vi "ControladorPIDparaSEIG.vi"() -> ()   [LabVIEW 2019]
uses:
  <resource>/objmgr/daqmx.rc
  <vilib>/addons/control/pid/NI_PID_pid.lvlib
  <vilib>/NI/Modbus Library/API/Wrapper/API Main.lvlib
  <vilib>/NI/Modbus Library/API/Master/Modbus Master.lvclass
  <vilib>/NI/Modbus Library/API/Wrapper/Create Serial Master.vi
  <vilib>/DAQmx/configure/timing.llb/DAQmx Timing (Sample Clock).vi
  <vilib>/DAQmx/create/channels.llb/DAQmx Create Channel (AI-Voltage-Basic).vi
  <vilib>/DAQmx/read.llb/DAQmx Read (Analog 2D DBL NChan NSamp).vi
  <vilib>/addons/control/pid/pid.llb/PID (DBL).vi
panel:
  in  "Tab Control":enum32{"Configuracion", "Datos"}(tab)=enum."Datos"
  in  "Valor máximo en la entrada":dbl=5.0 format="%0.2f"
  in  "Valor mínimo en la entrada":dbl=-5.0 format="%0.2f"
  in  "Modo de muestreo":i32(ring)=10123 items=["Finite Samples"=10178, "Continuous Samples"=10123, "Hardware Timed Single Point"=12522]
  in  "Muestras por canal":i32=500
  in  "Frecuencia de muetreo":dbl=2000.0 format="%0.2f"
  in  "VISA resource name":refnum<visa-resource-name>="COM3"
  in  "baud rate":u32=9600
  in  "unit ID":u8=17
  in  "physical channels":tag="myDAQ2/ai1, myDAQ2/ai0 "
  in  "number of samples per channel":i32=500
  out "dt out (s)":dbl=1e-05 format="%.3f"
  out "# pending remove":i32
  out "Ajuste VFD\n(Hz)":dbl=40.0 format="%#_4f"
  out "Voltage medido \n(Vrms)":dbl=0.3833916457369924 format="%#_4f"
  out "Actual Sample Rate":dbl=2000.0
  in  "Voltaje deseado\n(Vrms)":dbl=145.0 step=10.0
  in  "PID constantes":T1={"proportional gain (Kc)"=0.08, "integral time (Ti, min)"=0.0, "derivative time (Td, min)"=0.0} {"derivative time (Td, min)" format="%.3f"; "integral time (Ti, min)" format="%.3f"; "proportional gain (Kc)" format="%.3f"}
  out "Salida PID":dbl=5.0 format="%.2f"
  in  "Stop":bool
  out "Corriente Medida\n(Irms)":dbl=0.3833916457369924 format="%#_4f"
  out "Velocidad\nmedida (rpm)":i32
  out "Tension":cluster{"Vd":dbl, dbl}(graph) caption="Waveform Chart"
  out "Corriente":dbl(graph) caption="Waveform Chart"
  out "Velocidad":dbl(graph) caption="Waveform Chart"
  # "Modbus"
  # "Generador"
  # "Counter"
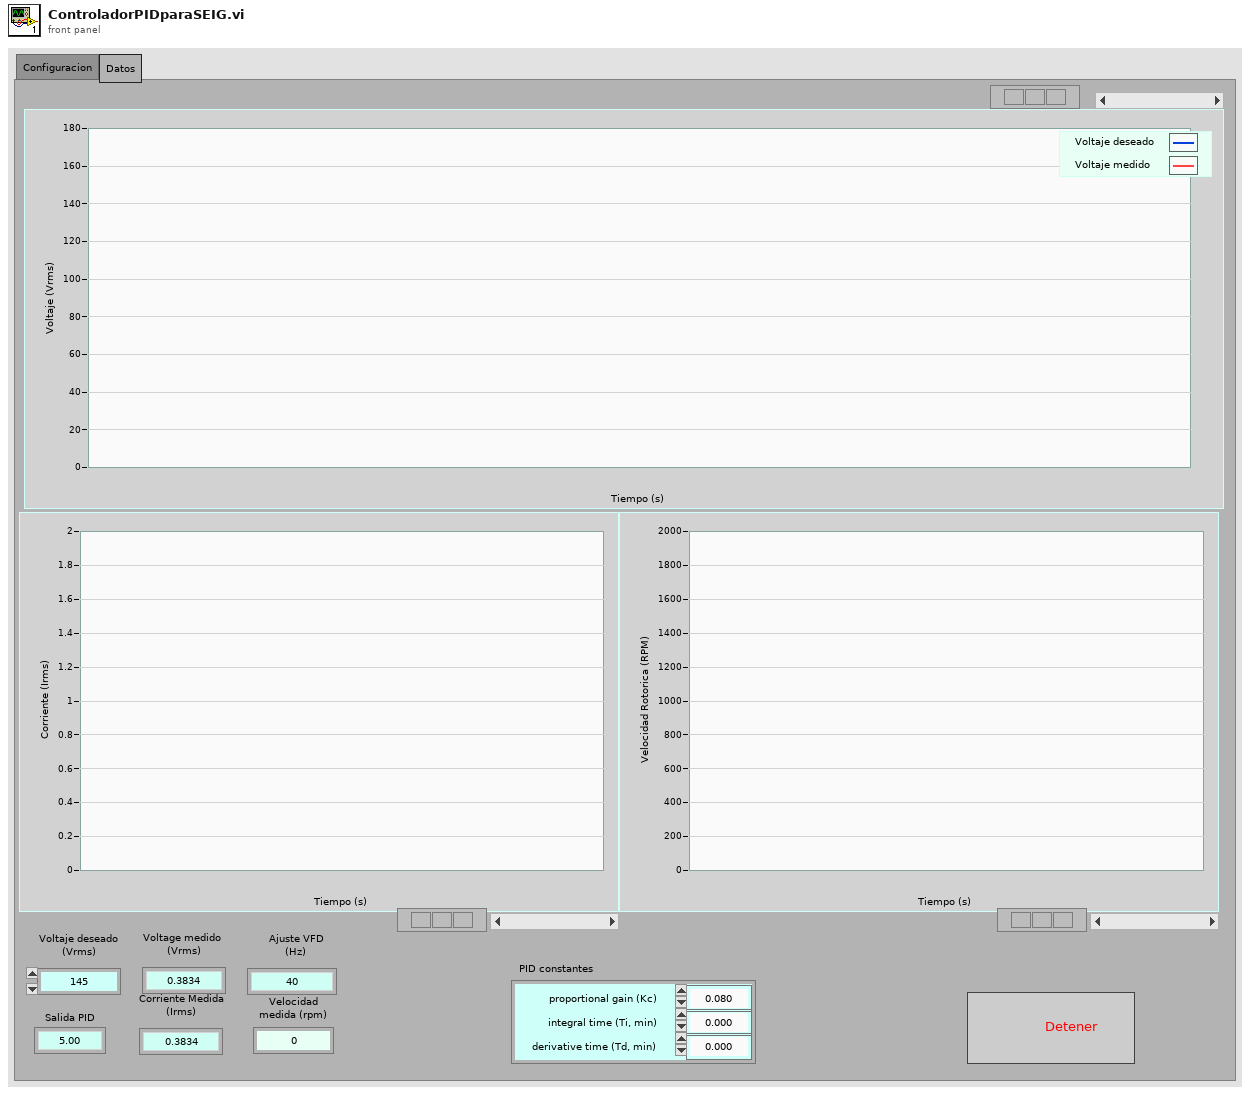
[diagram p1: front panel]
types:
  T1 = cluster{"proportional gain (Kc)":dbl, "integral time (Ti, min)":dbl, "derivative time (Td, min)":dbl}
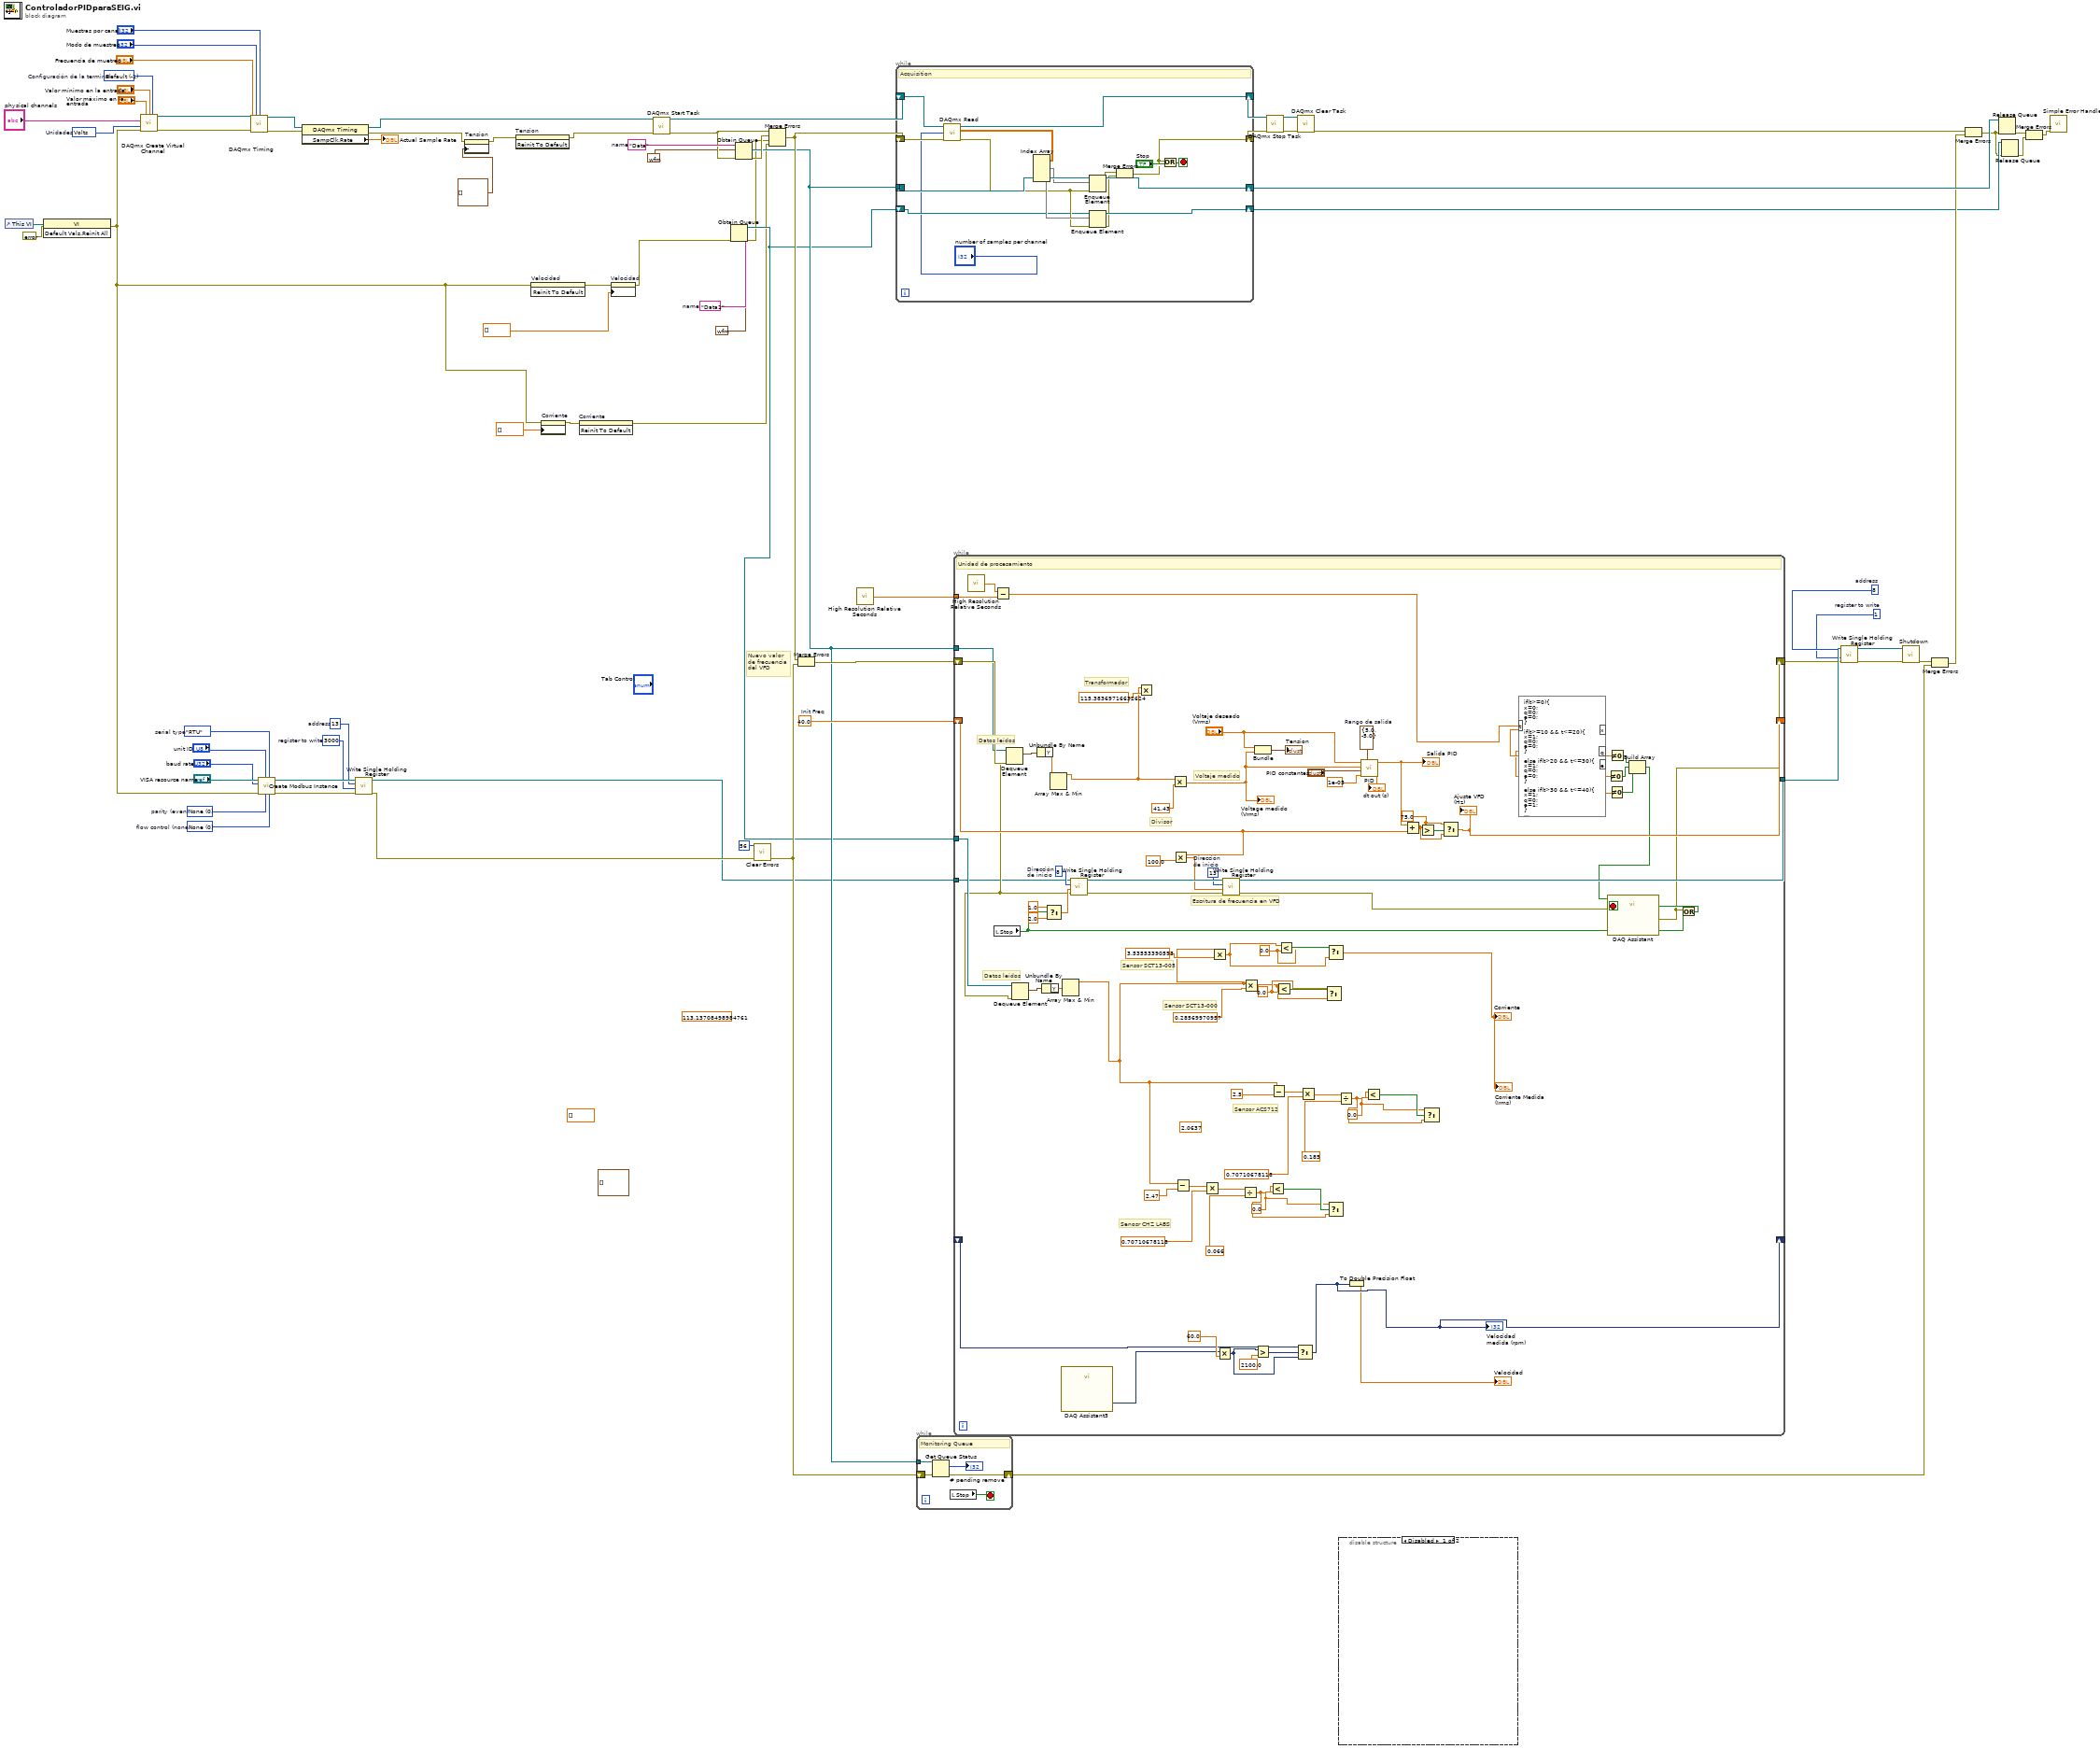
[diagram p0: block diagram]
diagram:
  (unwired) 113.13708498984761 ("y")
  (unwired) cluster{"Voltaje\ndeseado (Vrms)":dbl, dbl}[] [] ("History Data")
  (unwired) dbl[] [] ("History Data")
  w21 = "Data1"  # name
  w24 = u16 1  # register to write
  w25 = u16 8  # address
  w41 = u16 3000  # register to write
  w42 = u16 13  # address
  w47 = u16 0 items=["None", "XON/XOFF", "RTS/CTS", "XON/XOFF & RTS/CTS", "DTR/DSR", "XON/XOFF & DTR/DSR"]  # flow control (none)
  w48 = u16 0 items=["None", "Odd", "Even", "Mark", "Space"]  # parity (even)
  w49 = enum16{"RTU", "ASCII"}."RTU"  # serial type
  w52 = 40.0  # Init Freq
  w59 = "Data"  # name
  w72 = -1 items=["Default"=-1, "RSE"=10083, "NRSE"=10078, "Differential"=10106, "Pseudodifferential"=12529]  # Configuración de la terminal
  w75 = 10348 items=["Volts"=10348, "From Custom Scale"=10065]  # Unidades
  # "Nuevo valor\nde frecuencia\ndel VFD"
  n1 = control-ref of="This VI"() -> (w32:refnum<vi>)
  n2 = invoke class="VI" method="Default Vals.Reinit All"(reference=w32, error in=errorcluster {"status"=FALSE, "code"=0, "source"=""} ("error constant")) -> (error out=w7:errorcluster)  [unwired: 1 in, 2 out]
  n3 = call-poly <vilib>:"DAQmx Create Virtual Channel.vi"("maximum value"="Valor máximo en la entrada", "minimum value"="Valor mínimo en la entrada", "input terminal configuration"=w72, "physical channels"="physical channels", "units"=w75, "error in"=w7) -> ("task out"=w70:refnum<k21>, "error out"=w71:errorcluster)  [unwired: 8 in]
  n4 = call-poly <vilib>:"DAQmx Timing.vi"("task/channels in"=w70, "sample mode"="Modo de muestreo", "samples per channel"="Muestras por canal", "rate"="Frecuencia de muetreo", "error in"=w71) -> ("task out"=w61:refnum<k21>, "error out"=w60:errorcluster)  [unwired: 9 in]
  n5 = call-poly <vilib>:"Create Modbus Instance.vi"("flow control (none)"=w47, "serial type"=w49, "parity (even)"=w48, "unit ID"="unit ID", "error in"=w7, "baud rate"="baud rate", "VISA resource name"="VISA resource name") -> ("error out"=w44:errorcluster, "serial master instance"=w43:refnum<class "Modbus Master.lvclass">)  [unwired: 3 in]
  n6 = property class="DAQmx Timing"(reference=w61, error in=w60) -> (reference out=w23:refnum<k21>, error out=w3:errorcluster, "SampClk.Rate"=→"Actual Sample Rate":dbl)
  n7 = call-dynamic "Write Single Holding Register.vi"("error in"=w44, "register to write"=w41, "address"=w42, "Modbus master in"=w43) -> ("error out"=w2:errorcluster, "Modbus master out"=w1:refnum<class "Modbus Master.lvclass">)  [unwired: 6 in]
  n8 = property on="Tension" class="WFChart (strict)"(error in=w3, "History Data"=cluster{"Voltaje\ndeseado (Vrms)":dbl, dbl}[] []) -> (error out=w5:errorcluster)  [unwired: 1 in, 1 out]
  n9 = invoke on="Tension" class="WFChart (strict)" method="Reinit To Default"(error in=w5) -> (error out=w4:errorcluster)  [unwired: 2 in, 2 out]
  n10 = invoke on="Velocidad" class="WFChart (strict)" method="Reinit To Default"(error in=w7) -> (error out=w14:errorcluster)  [unwired: 2 in, 2 out]
  n11 = property on="Corriente" class="WFChart (strict)"(error in=w7, "History Data"=dbl[] []) -> (error out=w10:errorcluster)  [unwired: 1 in, 1 out]
  n12 = invoke on="Corriente" class="WFChart (strict)" method="Reinit To Default"(error in=w10) -> (error out=w9:errorcluster)  [unwired: 2 in, 2 out]
  n13 = property on="Velocidad" class="WFChart (strict)"(error in=w14, "History Data"=dbl[] []) -> (error out=w12:errorcluster)  [unwired: 1 in, 1 out]
  n14 = call <vilib>:"DAQmx Start Task.vi"("task/channels in"=w23, "error in"=w4) -> ("task out"=w67:refnum<k21>, "error out"=w58:errorcluster)  [unwired: 12 in]
  n15 = Obtain Queue(name (unnamed)=w21, element data type=waveform(dbl) {"t0"=timestamp(0 s since 1904-01-01), "dt"=0.0, "Y"=[]} ("data"), error in (no error)=w12) -> (queue out=w18:refnum<queue>, error out=w8:errorcluster)  [unwired: 2 in, 1 out]
  n16 = Obtain Queue(name (unnamed)=w59, element data type=waveform(dbl) {"t0"=timestamp(0 s since 1904-01-01), "dt"=0.0, "Y"=[]} ("data"), error in (no error)=w58) -> (queue out=w37:refnum<queue>, error out=w57:errorcluster)  [unwired: 2 in, 1 out]
  n17 = call <vilib>:"Clear Errors.vi"("error in (no error)"=w2, "specific error code to clear (0: all)"=56) -> ("error out"=w34:errorcluster)  [unwired: 4 in, 1 out]
  n18 = Merge Errors(w58, w57, w8, w9) -> (w56:errorcluster)
  n19 = Merge Errors(w56, w34) -> (w45:errorcluster)
  n20 = call <vilib>:"High Resolution Relative Seconds.vi"() -> ("relative seconds"=w22:dbl)
  n21 = while {
    shift-right: [w77] -> w64
    shift-left: w56 -> [w91]
    shift-right: [w89] -> w63
    shift-left: w67 -> [w90]
    tunnel: w37 -> [w88]
    shift-right: [w87] -> w38
    shift-left: _ -> [_]
    shift-right: [w80] -> w16
    shift-left: w18 -> [w81]
    stop <- w92 stop-if-true
    # "Acquisition"
    n22 = call-poly <vilib>:"DAQmx Read.vi"("task/channels in"=w90, "number of samples per channel"="number of samples per channel", "error in"=w91) -> ("task out"=w89:refnum<k21>, "data"=w85:dbl[][], "error out"=w82:errorcluster)  [unwired: 10 in]
    n23 = Index Array(array=w85) -> (element #1=w84:dbl[], element #2=w83:dbl[])  [unwired: 4 in]
    n24 = Enqueue Element(queue=w88, element=w84, error in (no error)=w82) -> (queue out=w87:refnum<queue>, error out=w79:errorcluster)  [unwired: 1 in, 1 out]
    n25 = Enqueue Element(queue=w81, element=w83, error in (no error)=w82) -> (queue out=w80:refnum<queue>, error out=w78:errorcluster)  [unwired: 1 in, 1 out]
    n26 = Merge Errors(w79, w78) -> (w77:errorcluster)
    n27 = Or(x=w77, y="Stop") -> (x .or. y?=w92:bool)
  }
  n28 = while {
    tunnel: w37 -> [w96]
    shift-right: [w94] -> w35
    shift-left: w34 -> [w97]
    stop <- w93 stop-if-true
    # "Monitoring Queue"
    n29 = Get Queue Status(queue=w96, error in (no error)=w97) -> (# pending remove=→"# pending remove":i32, error out=w94:errorcluster)  [unwired: 1 in, 6 out]
    n30 = local read "Stop"() -> (w93:bool)
  }
  n31 = while {
    tunnel: w37 -> [w179]
    shift-right: [w153] -> w28
    shift-left: w45 -> [w180]
    shift-right: [w157] -> _
    shift-left: w52 -> [w144]
    tunnel: [w164] -> w29
    tunnel: w22 -> [w146]
    tunnel: w18 -> [w141]
    shift-right: [w134] -> _
    shift-left: _ -> [w133]
    tunnel: w1 -> [w102]
    stop <- w172 stop-if-true
    w114 = 0.0 ("y")
    w123 = 0.0 ("y")
    w127 = 0.0 ("y")
    (unwired) 2.0637 ("y")
    w107 = 0.0 ("y")
    w156 = 75.0 ("y")
    w166 = u16 13  # Dirección de inicio
    w169 = u16 8  # Dirección de inicio
    w177 = cluster{"output high":dbl, "output low":dbl} {"output high"=5.0, "output low"=-5.0}  # Rango de salida
    # "Divisor"
    # "Transformador"
    # "Sensor ACS712"
    # "Senosr CHZ LABS"
    # "Sensor SCT13-005"
    # "Sensor SCT13-000"
    # "Datos leídos"
    # "Escritura de frecuencia en VFD"
    # "Voltaje medido"
    # "Datos leídos"
    # "Unidad de procesamiento"
    n32 = call <vilib>:"High Resolution Relative Seconds.vi"() -> ("relative seconds"=w147:dbl)
    n33 = local read "Stop"() -> (w171:bool)
    n34 = Subtract(x=w147, y=w146) -> (x-y=w145:dbl)
    n35 = Dequeue Element(queue=w179, error in (no error)=w180) -> (element=w163:waveform(dbl), error out=w140:errorcluster)  [unwired: 1 in, 2 out]
    n36 = Dequeue Element(queue=w141, error in (no error)=w140) -> (element=w142:waveform(dbl))  [unwired: 1 in, 3 out]
    n37 = Unbundle By Name(w163) -> ("Y"=w176:dbl[])
    n38 = Unbundle By Name(w142) -> ("Y"=w143:dbl[])
    n39 = Select(t=1.0, s=w171, f=2.0 ("t")) -> (s? t:f=w170:dbl)
    n40 = Array Max & Min(array=w176) -> (max value=w98:dbl)  [unwired: 3 out]
    n41 = call "DAQ Assistant3"() -> ("data"=w135:dynamicdata)  [unwired: 17 in, 2 out]
    n42 = Array Max & Min(array=w143) -> (max value=w101:dbl)  [unwired: 3 out]
    n43 = call-dynamic "Write Single Holding Register.vi"("error in"=w140, "register to write"=w170, "address"=w169, "Modbus master in"=w102) -> ("error out"=w167:errorcluster, "Modbus master out"=w168:refnum<class "Modbus Master.lvclass">)  [unwired: 6 in]
    n44 = Multiply(x=w98, y=115.38369716632624) -> ()  [unwired: 1 out]
    n45 = Multiply(x=w98, y=41.43) -> (x*y=w175:dbl)
    "Voltage medido \n(Vrms)" <- w175
    n46 = Multiply(x=w144, y=100.0) -> (x*y=w165:dbl)
    n47 = Subtract(x=w101, y=2.47) -> (x-y=w111:dbl)
    n48 = Multiply(x=w111, y=0.70710678118) -> (x*y=w110:dbl)
    n49 = Multiply(x=w101, y=3.53553390593) -> (x*y=w106:dbl)
    n50 = Multiply(x=w135, y=60.0) -> (x*y=w136:dynamicdata)
    n51 = call-dynamic "Write Single Holding Register.vi"("error in"=w167, "register to write"=w165, "address"=w166, "Modbus master in"=w168) -> ("error out"=w154:errorcluster, "Modbus master out"=w164:refnum<class "Modbus Master.lvclass">)  [unwired: 6 in]
    n52 = Divide(x=w110, y=0.066) -> (x/y=w108:dbl)
    n53 = Multiply(x=w101, y=0.28569970957) -> (x*y=w125:dbl)
    n54 = Bundle("Voltaje deseado\n(Vrms)"="Voltaje deseado\n(Vrms)", w175) -> (→"Tension":cluster{"Voltaje deseado\n(Vrms)":dbl, dbl})  [unwired: 1 in]
    n55 = Greater?(x=w136, y=2100.0) -> (0:w132:dynamicdata)
    n56 = Less?(x=w108, y=w114) -> (x < y?=w115:bool)
    n57 = Subtract(x=w101, y=2.5) -> (x-y=w120:dbl)
    n58 = Less?(x=w125, y=w127) -> (x < y?=w128:bool)
    n59 = Less?(x=w106, y=w107) -> (x < y?=w131:bool)
    n60 = Select(t=w133, s=w132, f=w136) -> (s? t:f=w134:dynamicdata)
    "Velocidad\nmedida (rpm)" <- w134
    n61 = Multiply(x=w120, y=0.70710678118) -> (x*y=w119:dbl)
    n62 = Select(t=w127, s=w128, f=w125) -> ()  [unwired: 1 out]
    n63 = Select(t=w107, s=w131, f=w106) -> (s? t:f=→"Corriente Medida\n(Irms)" →"Corriente":dbl)
    n64 = Select(t=w114, s=w115, f=w108) -> ()  [unwired: 1 out]
    n65 = Divide(x=w119, y=0.185) -> (x/y=w117:dbl)
    n66 = To Double Precision Float(number=w134) -> (double precision float=→"Velocidad":dbl)
    n67 = call-poly <vilib>:"PID.vi"("output range"=w177, "dt (s)"=1e-05, "PID gains"="PID constantes", "process variable"=w175, "setpoint"="Voltaje deseado\n(Vrms)") -> ("dt out (s)"=→"dt out (s)":dbl, "output"=w178:dbl)  [unwired: 5 in]
    "Salida PID" <- w178
    n68 = Less?(x=w117, y=w123) -> (x < y?=w124:bool)
    n69 = Add(x=w178, y=w144) -> (x+y=w155:dbl)
    n70 = Greater?(x=w155, y=w156) -> (0:w158:bool)
    n71 = Select(t=w123, s=w124, f=w117) -> ()  [unwired: 1 out]
    n72 = Select(t=w156, s=w158, f=w155) -> (s? t:f=w157:dbl)
    "Ajuste VFD\n(Hz)" <- w157
    n73 = formula code="if(t>=0){\nx=0;\nq=0;\ne=0;\n}\n\nif(t>=10 && t<=20){\nx=1;\nq=0;\ne=0;\n}\n\nelse if(t>20 && t<=30){\nx=1;\nq=0;\ne=0;\n}\n\nelse if(t>30 && t<=40){\nx=1;\nq=0;\ne=1;\n}\n\nelse if(t>40 && t<=50){\nx=0;\nq=0;\ne=1;\n}\n\nelse{\nx=0;\nq=0;\ne=1;\n}"("t"=w145) -> ("x"=w152:dbl, "q"=w151:dbl, "e"=w103:dbl)
    n74 = Not Equal To 0?(x=w151) -> (x != 0?=w149:bool)
    n75 = Not Equal To 0?(x=w103) -> (x != 0?=w104:bool)
    n76 = Not Equal To 0?(x=w152) -> (x != 0?=w150:bool)
    n77 = Build Array(w150, w149, w104) -> (w148:bool[])
    n78 = call "DAQ Assistant"("data"=w148, "error in"=w154) -> ("error out"=w153:errorcluster)  [unwired: 16 in, 1 out]
    n79 = Or(x=w153, y=w171) -> (x .or. y?=w172:bool)
  }
  n80 = call <vilib>:"DAQmx Stop Task.vi"("task/channels in"=w63, "error in"=w64) -> ("task out"=w66:refnum<k21>, "error out"=w65:errorcluster)  [unwired: 12 in]
  n81 = call <vilib>:"DAQmx Clear Task.vi"("task in"=w66, "error in"=w65) -> ("error out"=w62:errorcluster)  [unwired: 13 in]
  n82 = disable-structure shown="Disabled" {
    frame Disabled {
    }
    frame Enabled {
    }
  }
  n83 = call-dynamic "Write Single Holding Register.vi"("error in"=w28, "register to write"=w24, "address"=w25, "Modbus master in"=w29) -> ("error out"=w26:errorcluster, "Modbus master out"=w27:refnum<class "Modbus Master.lvclass">)  [unwired: 6 in]
  n84 = call-dynamic "Shutdown.vi"("error in"=w26, "Modbus master in"=w27) -> ("error out"=w40:errorcluster)  [unwired: 9 in]
  n85 = Merge Errors(w40, w35) -> (w36:errorcluster)
  n86 = Merge Errors(w62, w36) -> (w15:errorcluster)
  n87 = Release Queue(queue=w38, error in (no error)=w15) -> (error out=w39:errorcluster)  [unwired: 1 in, 2 out]
  n88 = Release Queue(queue=w16, error in (no error)=w15) -> (error out=w17:errorcluster)  [unwired: 1 in, 2 out]
  n89 = Merge Errors(w39, w17) -> (w55:errorcluster)
  n90 = call <vilib>:"Simple Error Handler.vi"("error in (no error)"=w55) -> ()  [unwired: 4 in, 5 out]
